vi "SID_filter.vi"(5 "sampling info":cluster{"Fs":dbl, "#s":i32}={"Fs"=44100.0, "#s"=50}, 6 "reset":bool=TRUE, 7 "filter":T2={"freq"=70.6, "res"=240.0, "HP"=FALSE, "BP"=FALSE, "LP"=TRUE, "VC1"=TRUE, "VC2"=TRUE, "VC3"=TRUE, "vol"=1.0} {"vol" format="%0.2f"; "res" format="%0.2f"; "freq" format="%0.2f"}, 9 "VC3":dbl[](array[numeric]), 10 "VC2":dbl[](array[numeric]), 11 "VC1":dbl[](array[numeric])) -> (3 "out":dbl[](array[numeric]))   [LabVIEW 2018]
uses:
  SID_filter_reg.ctl
  <vilib>/Analysis/3filter.llb/Filter Passband Type.ctl
  <vilib>/Analysis/3filter.llb/Chebyshev Filter (DBL).vi
  <vilib>/Analysis/NI_AALBase.lvlib
panel:
  out "filter type":T1
  out "freq":dbl
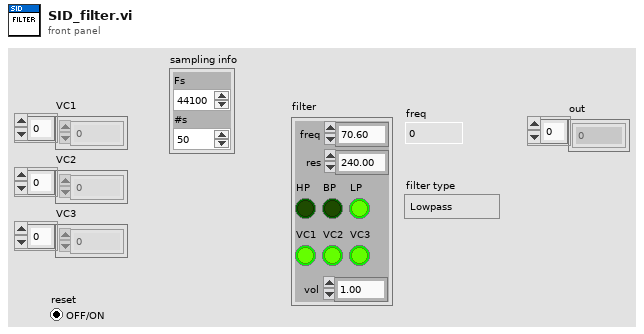
[diagram p1: front panel]
types:
  T1 = typedef "NI_AALBase.lvlib/Filter Passband Type.ctl" = enum32{"Lowpass", "Highpass", "Bandpass", "Bandstop"}
  T2 = typedef "SID_filter_reg.ctl" = cluster{"freq":dbl, "res":dbl, "HP":bool, "BP":bool, "LP":bool, "VC1":bool, "VC2":bool, "VC3":bool, "vol":dbl}
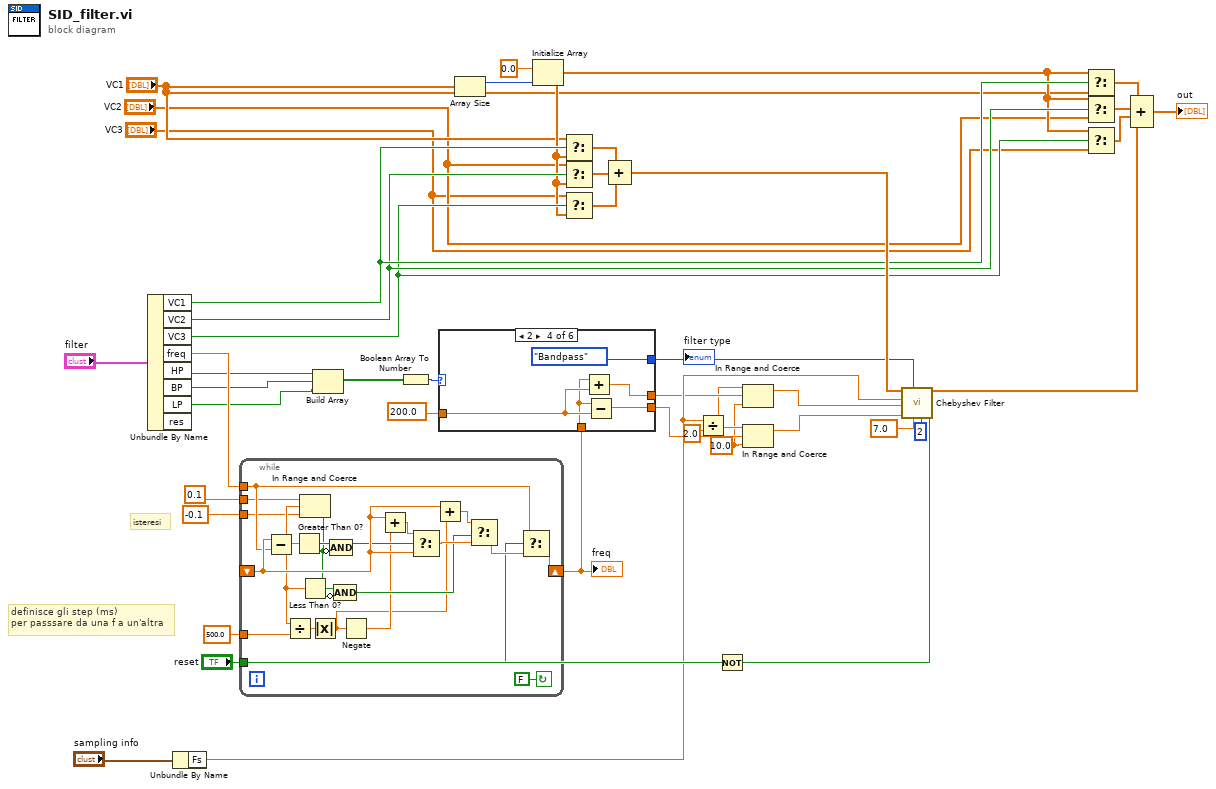
[diagram p0: block diagram]
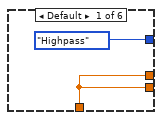
[diagram p2: hidden frame]
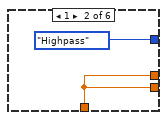
[diagram p3: hidden frame]
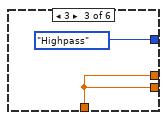
[diagram p4: hidden frame]
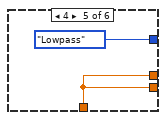
[diagram p5: hidden frame]
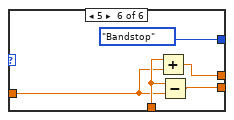
[diagram p6: hidden frame]
diagram:
  w1 = 10.0 ("lower limit")
  # "isteresi"
  # "definisce gli step (ms)\nper passsare da una f a un'altra"
  n1 = Unbundle By Name("filter") -> ("VC1"=w29:bool, "VC2"=w28:bool, "VC3"=w27:bool, "freq"=w43:dbl, "HP"=w21:bool, "BP"=w20:bool, "LP"=w19:bool)  [unwired: 1 out]
  n2 = Unbundle By Name("sampling info") -> ("Fs"=w6:dbl)
  n3 = while {
    tunnel: w43 -> [w56]
    shift-right: [w54] -> w11
    shift-left: _ -> [w61]
    tunnel: "reset" -> [w53]
    tunnel: 0.1 ("x") -> [w47]
    tunnel: -0.1 ("x") -> [w49]
    tunnel: 500.0 ("y") -> [w45]
    stop <- FALSE continue-if-true
    n4 = Subtract(x=w61, y=w56) -> (x-y=w51:dbl)
    n5 = Divide(x=w51, y=w45) -> (x/y=w48:dbl)
    n6 = Greater Than 0?(x=w51) -> (x > 0?=w65:bool)
    n7 = In Range and Coerce(upper limit=w47, x=w51, lower limit=w49) -> (In Range?=w57:bool)  [unwired: 1 out]
    n8 = Less Than 0?(x=w51) -> (x < 0?=w59:bool)
    n9 = Absolute Value(x=w48) -> (abs(x)=w46:dbl)
    n10 = Compound Arithmetic op=AND(w65, invert w57) -> (w60:bool)
    n11 = Compound Arithmetic op=AND(w59, invert w57) -> (w58:bool)
    n12 = Negate(x=w46) -> (-x=w50:dbl)
    n13 = Add(x=w61, y=w50) -> (x+y=w64:dbl)
    n14 = Select(t=w64, s=w60, f=w61) -> (s? t:f=w62:dbl)
    n15 = Add(x=w61, y=w46) -> (x+y=w63:dbl)
    n16 = Select(t=w63, s=w58, f=w62) -> (s? t:f=w55:dbl)
    n17 = Select(t=w56, s=w53, f=w55) -> (s? t:f=w54:dbl)
  }
  "freq" <- w11
  n18 = Build Array(w21, w20, w19) -> (w18:bool[])
  n19 = Boolean Array To Number(Boolean array=w18) -> (number=w17:u32)
  n20 = case shown="2" w17 {
    tunnel: [Filter_Passband_Type."Highpass" ("filter type") Filter_Passband_Type."Highpass" ("filter type") Filter_Passband_Type."Highpass" ("filter type") Filter_Passband_Type."Bandpass" ("filter type") Filter_Passband_Type."Lowpass" ("filter type") Filter_Passband_Type."Bandstop" ("filter type")] -> w16
    tunnel: w11 -> [w66 w68 w70 w74 w77 w82]
    tunnel: [w66 w68 w70 w72 w77 w79] -> w5
    tunnel: [w66 w68 w70 w73 w77 w80] -> w8
    tunnel: 200.0 ("ripple(dB)") -> [_ _ _ w75 _ w81]
    frame Default {
    }
    frame 1 {
    }
    frame 3 {
    }
    frame 2 {
      n21 = Add(x=w74, y=w75) -> (x+y=w72:dbl)
      n22 = Subtract(x=w74, y=w75) -> (x-y=w73:dbl)
    }
    frame 4 {
    }
    frame 5 {
      n23 = Add(x=w82, y=w81) -> (x+y=w79:dbl)
      n24 = Subtract(x=w82, y=w81) -> (x-y=w80:dbl)
    }
  }
  "filter type" <- w16
  n25 = Array Size(array="VC1") -> (size(s)=w40:i32)
  n26 = Initialize Array(0.0 ("element"), w40) -> (w26:dbl[])
  n27 = Select(t="VC1", s=w29, f=w26) -> (s? t:f=w38:dbl[])
  n28 = Select(t="VC2", s=w28, f=w26) -> (s? t:f=w37:dbl[])
  n29 = Select(t="VC3", s=w27, f=w26) -> (s? t:f=w36:dbl[])
  n30 = Compound Arithmetic op=ADD(w38, w37, w36) -> (w35:dbl[])
  n31 = Divide(x=w6, y=2.0 ("lower limit")) -> (x/y=w2:dbl)
  n32 = Not(x="reset") -> (.not. x?=w12:bool)
  n33 = In Range and Coerce(upper limit=w2, x=w5, lower limit=w1) -> (coerced(x)=w4:dbl)  [unwired: 1 out]
  n34 = In Range and Coerce(upper limit=w2, x=w8, lower limit=w1) -> (coerced(x)=w7:dbl)  [unwired: 1 out]
  n35 = call-poly <vilib>:"Chebyshev Filter.vi"("init/cont (init:F)"=w12, "order"=2, "ripple(dB)"=7.0, "filter type"=w16, "low cutoff freq: fl"=w7, "high cutoff freq: fh"=w4, "sampling freq: fs"=w6, "X"=w35) -> ("Filtered X"=w31:dbl[])  [unwired: 2 in, 1 out]
  n36 = Select(t=w26, s=w29, f="VC1") -> (s? t:f=w32:dbl[])
  n37 = Select(t=w26, s=w28, f="VC2") -> (s? t:f=w33:dbl[])
  n38 = Select(t=w26, s=w27, f="VC3") -> (s? t:f=w34:dbl[])
  n39 = Compound Arithmetic op=ADD(w32, w33, w34, w31) -> (→"out":dbl[])
